vi "gRPC Client Cache FGV Impl.vi"(8 "error in":errorcluster, 9 "unique id in":u64, 10 "action":T3, 11 "vi references in":T1) -> (0 "error out":errorcluster, 1 "unique id out":u64, 2 "grpc client id":T2)   [LabVIEW 2020, in "MeasurementLink Discovery V1.lvlib"]
uses:
  MeasurementLink Discovery V1.lvlib
  TypeDefs/gRPC Client Cache FGV Action.ctl
  <vilib>/gRPC/LabVIEW gRPC Library/Shared/grpcId.ctl
  TypeDefs/gRPC Client Cache VI References.ctl
  <vilib>/gRPC/LabVIEW gRPC Library/grpc-lvsupport-release.lvlib
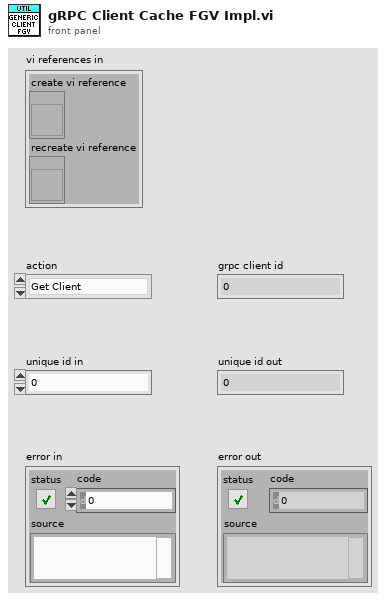
[diagram p1: front panel]
types:
  T1 = typedef "MeasurementLink Discovery V1.lvlib/gRPC Client Cache VI References.ctl" = cluster{"create vi reference":refnum<vi>, "recreate vi reference":refnum<vi>}
  T2 = typedef "grpc-lvsupport-release.lvlib/grpcId.ctl" = u64
  T3 = typedef "MeasurementLink Discovery V1.lvlib/gRPC Client Cache FGV Action.ctl" = enum16{"Get Client", "Recreate Client"}
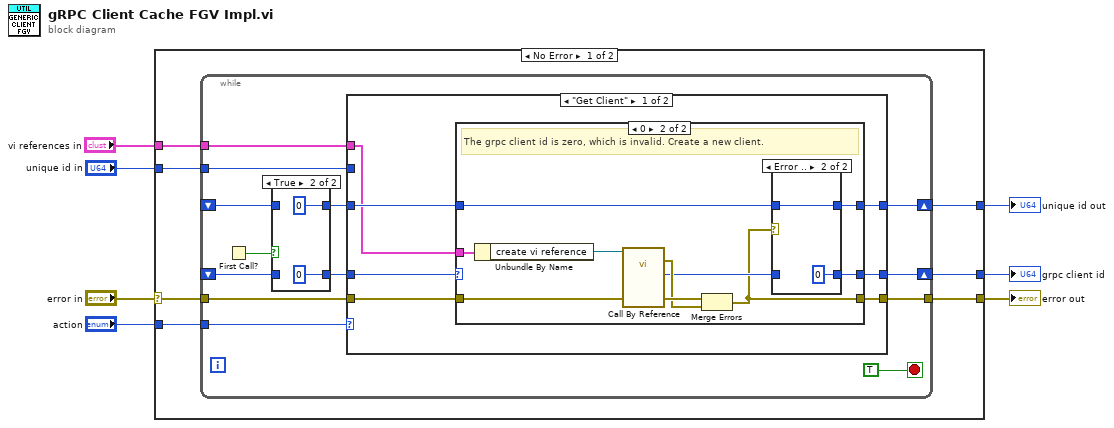
[diagram p0: block diagram]
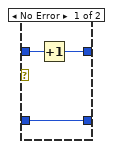
[diagram p4: hidden frame]
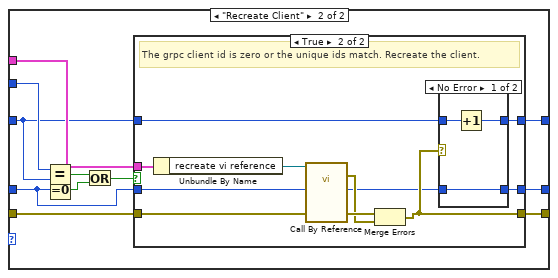
[diagram p5: hidden frame]
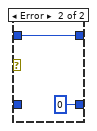
[diagram p7: hidden frame]
diagram:
  n1 = case shown="No Error" "error in" {
    selector: "error in" -> [w13 w87]
    tunnel: [w12 w87] -> w7
    tunnel: "action" -> [w14 _]
    tunnel: [w11 _] -> w6
    tunnel: [w10 _] -> w5
    tunnel: "unique id in" -> [w9 _]
    tunnel: "vi references in" -> [w8 _]
    frame No Error {
      n2 = while {
        tunnel: w14 -> [w26]
        tunnel: w13 -> [w25]
        tunnel: [w24] -> w12
        shift-right: [w23] -> w11
        shift-left: _ -> [w21]
        shift-right: [w17] -> w10
        shift-left: _ -> [w19]
        tunnel: w9 -> [w16]
        tunnel: w8 -> [w15]
        stop <- TRUE stop-if-true
        n3 = First Call?() -> (First Call?: T/F=w22:bool)
        n4 = case shown="True" w22 {
          tunnel: w21 -> [w29 _]
          tunnel: [w29 T2 0 ("gRPC ID out")] -> w20
          tunnel: w19 -> [w28 _]
          tunnel: [w28 u64 0] -> w18
          frame False {
          }
          frame True {
          }
        }
        n5 = case shown="\"Get Client\"" w26 {
          tunnel: w25 -> [w35 w66]
          tunnel: [w38 w67] -> w24
          tunnel: [w37 w64] -> w23
          tunnel: w20 -> [w36 w57]
          tunnel: w18 -> [w34 w62]
          tunnel: [w33 w61] -> w17
          tunnel: w16 -> [_ w65]
          tunnel: w15 -> [w32 w63]
          frame "Get Client" {
            n6 = case shown="0" w36 {
              selector: w36 -> [w41 _]
              tunnel: w35 -> [w40 w50]
              tunnel: [w40 w42] -> w38
              tunnel: [w41 w45] -> w37
              tunnel: w34 -> [w39 w44]
              tunnel: [w39 w43] -> w33
              tunnel: w32 -> [_ w49]
              frame Default {
                # "The grpc client id is non-zero. As far as we know, it is valid, so return it."
              }
              frame 0 {
                # "The grpc client id is zero, which is invalid. Create a new client."
                n7 = Unbundle By Name(w49) -> ("create vi reference"=w51:refnum<vi>)
                n8 = call-by-ref "?"(reference=w51, "error in"=w50) -> (error out=w47:errorcluster, 0:"error out"=w48:errorcluster, "grpc client id"=w46:T2)  [unwired: 10 in, 1 out]
                n9 = Merge Errors(w48, w47) -> (w42:errorcluster)
                n10 = case shown="Error .." w42 {
                  tunnel: w44 -> [w54 w55]
                  tunnel: [w53 w55] -> w43
                  tunnel: w46 -> [w52 _]
                  tunnel: [w52 T2 0 ("grpc client id out")] -> w45
                  frame No Error {
                    n11 = Increment(x=w54) -> (x+1=w53:u64)
                  }
                  frame Error {
                  }
                }
              }
            }
          }
          frame "Recreate Client" {
            n12 = Equal?(x=w65, y=w62) -> (x = y?=w60:bool)
            n13 = Equal To 0?(x=w57) -> (x = 0?=w58:bool)
            n14 = Or(x=w60, y=w58) -> (x .or. y?=w59:bool)
            n15 = case shown="True" w59 {
              tunnel: w57 -> [w69 w79]
              tunnel: [w70 w75] -> w67
              tunnel: w66 -> [w70 w78]
              tunnel: [w69 w71] -> w64
              tunnel: w63 -> [_ w81]
              tunnel: w62 -> [w68 w74]
              tunnel: [w68 w73] -> w61
              frame False {
                # "The grpc client id is non-zero and the unique ids don't match. The client has already been recreated, so just return it."
              }
              frame True {
                # "The grpc client id is zero or the unique ids match. Recreate the client."
                n16 = Unbundle By Name(w81) -> ("recreate vi reference"=w80:refnum<vi>)
                n17 = call-by-ref "?"(reference=w80, "error in"=w78, "grpc client id in"=w79) -> (error out=w76:errorcluster, 0:"error out"=w77:errorcluster, "grpc client id out"=w72:T2)  [unwired: 9 in, 1 out]
                n18 = Merge Errors(w77, w76) -> (w75:errorcluster)
                n19 = case shown="No Error" w75 {
                  tunnel: w74 -> [w84 w86]
                  tunnel: [w83 w86] -> w73
                  tunnel: w72 -> [w82 _]
                  tunnel: [w82 T2 0 ("grpc client id out")] -> w71
                  frame No Error {
                    n20 = Increment(x=w84) -> (x+1=w83:u64)
                  }
                  frame Error {
                  }
                }
              }
            }
          }
        }
      }
    }
    frame Error {
    }
  }
  "error out" <- w7
  "grpc client id" <- w6
  "unique id out" <- w5
